vi "Send_command2.vi"(10 "String":string, 11 "VISA Refnum in":refnum<visa-resource-name>) -> (2 "string":string, 3 "VISA Refnum out":refnum<visa-resource-name>)   [LabVIEW 2013]
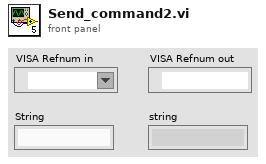
[diagram p1: front panel]
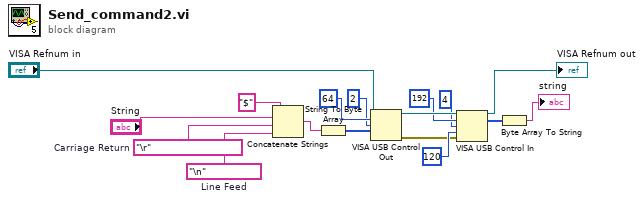
[diagram p0: block diagram]
diagram:
  w1 = "\n"  # Line Feed
  w2 = "\r"  # Carriage Return
  n1 = Concatenate Strings("$", "String", w2, w1) -> (w13:string)
  n2 = String To Byte Array(string=w13) -> (unsigned byte array=w10:u8[])
  n3 = VISA USB Control Out(0:"VISA Refnum in", 5:i16 64 ("request type"), 7:i16 2 ("request"), 9:w10) -> (4:w9:refnum<visa-resource-name>, 15:w8:errorcluster)  [unwired: 1 in, 2 out]
  n4 = VISA USB Control In(0:w9, 5:i16 192 ("request type"), 7:i16 4 ("request"), 9:u16 120 ("length (0)"), 11:w8) -> (4:→"VISA Refnum out":refnum<visa-resource-name>, 6:w5:u8[])  [unwired: 3 out]
  n5 = Byte Array To String(unsigned byte array=w5) -> (string=→"string":string)
